vi "Write tour.vi"(8 "error in (no error)":errorcluster, 11 "Completed tour paragraph":string) -> (0 "error out":errorcluster)   [LabVIEW 2018, in "app_log.lvlib"]
doc: "Writes (appends) a knight tour to the log file."
uses:
  app_log.lvlib
  text_file/text_file.lvlib
panel:
  # "Development\ncontrols/indicators useful for development and testing, but which are not outputs of the VI"
  # "Input\nInputs to the VI"
  # "Output\nOutputs of the VI"
  # "Description\n\nBlank VI with error handling case. \n\nSummarize the use of this VI in this space."
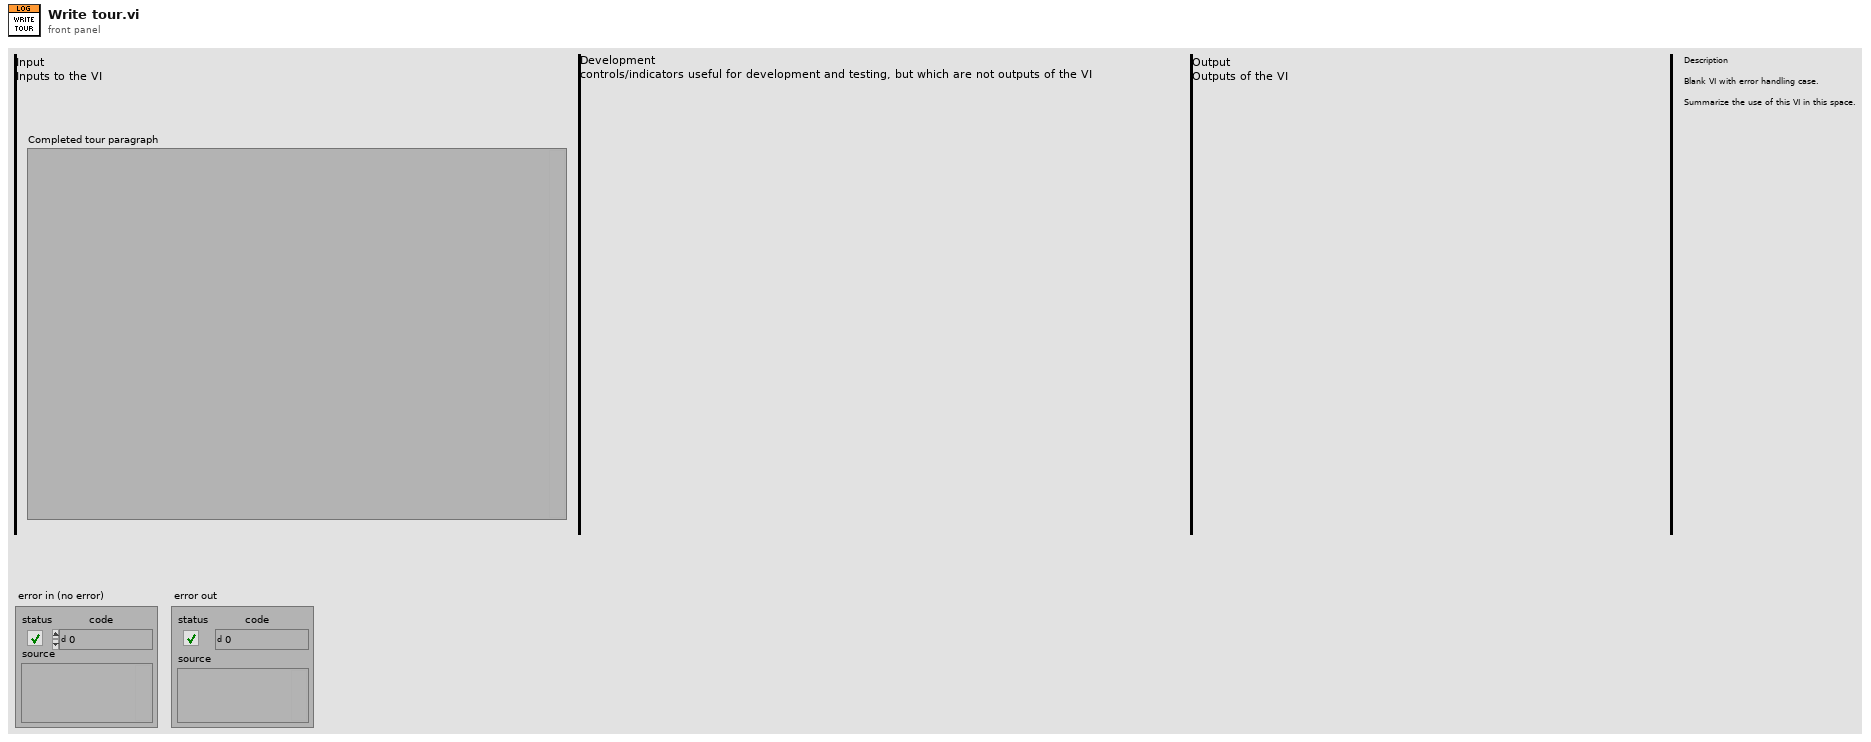
[diagram p1: front panel]
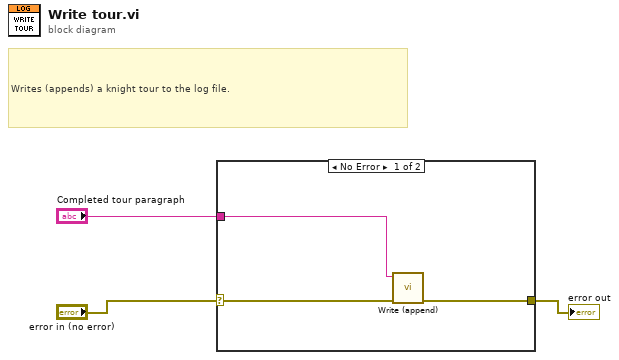
[diagram p0: block diagram]
diagram:
  # "Writes (appends) a knight tour to the log file."
  n1 = case shown="No Error" "error in (no error)" {
    selector: "error in (no error)" -> [w5 w7]
    tunnel: [w6 w7] -> w2
    tunnel: "Completed tour paragraph" -> [w4 _]
    frame No Error {
      n2 = call "Write (append).vi"("error in (no error)"=w5, "Write (append) this text to the file"=w4) -> ("error out"=w6:errorcluster)  [unwired: 9 in]
    }
    frame Error {
    }
  }
  "error out" <- w2
